vi "ICM aU8.vi"(11 "String In":string) -> (1 "Value U8":u8, 2 "Value":dbl, 3 "String Out":string)   [LabVIEW 2024]
doc: "ICM aU8.vi\n\n This VI is used to parse binary data that contains a U8 integer.\n\nThis VI was original part of the OSDS system.\n\nInstrument Communication Module Version 1.0\nSeptember, 2017 Original Code Consulting David Thomson\n www.originalcode.com"
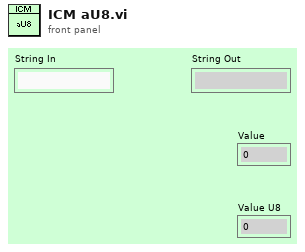
[diagram p1: front panel]
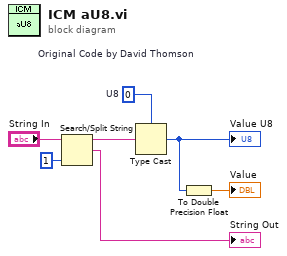
[diagram p0: block diagram]
diagram:
  w5 = u8 0  # U8
  n1 = Search/Split String(string="String In", offset (0)=1) -> (substring before match=w1:string, match + rest of string=→"String Out":string)  [unwired: 2 out]
  n2 = Type Cast "Original Code by David Thomson"(type=w5, x=w1) -> (*(type *) &x=w3:u8)
  "Value U8" <- w3
  n3 = To Double Precision Float(number=w3) -> (double precision float=→"Value":dbl)
